vi "VisionOnSWMap5LabModifiedOne.vi"(0 "SWMap In":i32[][](array[numeric]), 11 "Image Pixels":u32[][](array[numeric])) -> (4 "SWMap Out":i32[][](array[numeric]))   [LabVIEW 2014]
panel:
  out "test3":dbl
  out "test2":dbl
  out "test1":dbl
  # "Vision On SWMap"
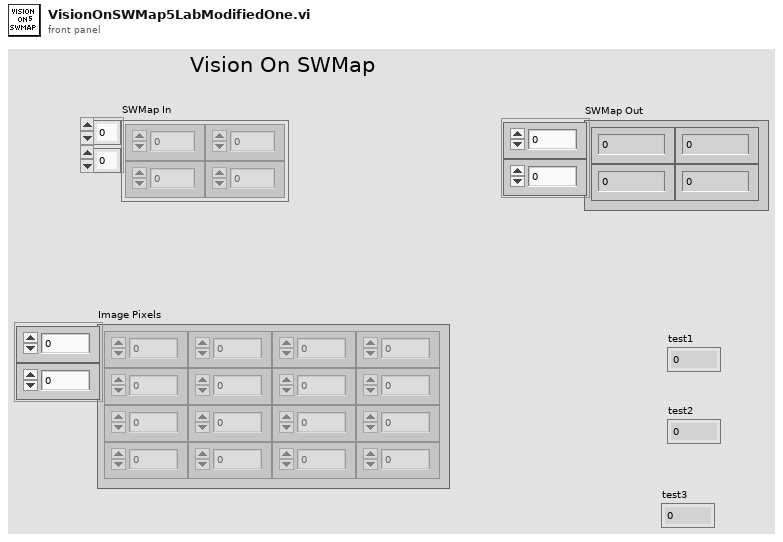
[diagram p1: front panel]
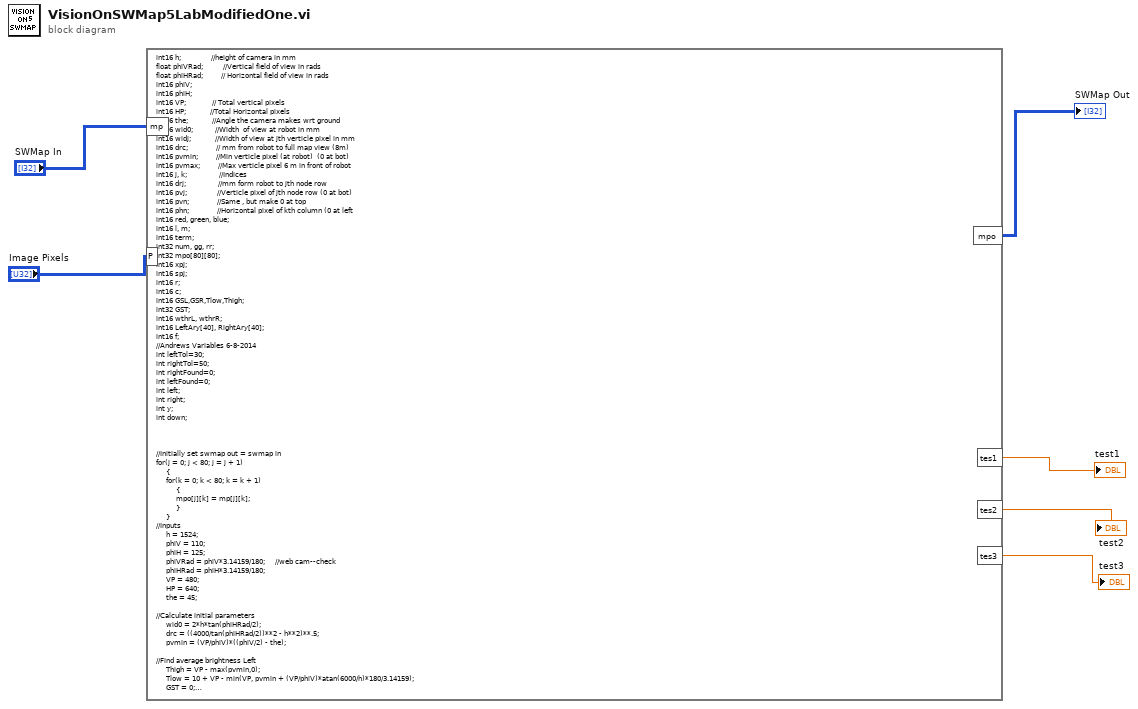
[diagram p0: block diagram]
diagram:
  n1 = formula code="int16 h;               //height of camera in mm\nfloat phiVRad;          //Vertical field of view in rads\nfloat phiHRad;         // Horizontal field of view in rads\nint16 phiV;\nint16 phiH;\nint16 VP;             // Total vertical pixels\nint16 HP;            //Total Horizontal pixels\nint16 the;            //Angle the camera makes wrt ground\nint16 wid0;           //Width  of view at robot in mm\nint16 widj;            //Width of view at jth verticle pixel in mm\nint16 drc;              // mm from robot to full map view (8m)\nint16 pvmin;         //Min verticle pixel (at robot)  (0 at bot)\nint16 pvmax;         //Max verticle pixel 6 m in front of robot\nint16 j, k;                //Indices\nint16 drj;                //mm form robot to jth node row\nint16 pvj;               //Verticle pixel of jth node row (0 at bot)\nint16 pvn;              //Same , but make 0 at top\nint16 phn;              //Horizontal pixel of kth column (0 at left\nint16 red, green, blue;\nint16 l, m;\nint16 term;\nint32 num, gg, rr;\nint32 mpo[80][80];\nint16 xpj;\nint16 spj;\nint16 r;\nint16 c;\nint16 GSL,GSR,Tlow,Thigh;\nint32 GST;\nint16 wthrL, wthrR;\nint16 LeftAry[40], RightAry[40];\nint16 f;\n//Andrews Variables 6-8-2014\nint leftTol=30;\nint rightTol=50;\nint rightFound=0;\nint leftFound=0;\nint left;\nint right;\nint y;\nint down;\n\n\n\n//Initially set swmap out = swmap in\nfor(j = 0; j < 80; j = j + 1)\n     {\n     for(k = 0; k < 80; k = k + 1)\n          {\n          mpo[j][k] = mp[j][k];\n          }\n     }\n//Inputs\n     h = 1524;\n     phiV = 110;\n     phiH = 125;\n     phiVRad = phiV*3.14159/180;     //web cam--check\n     phiHRad = phiH*3.14159/180;\n     VP = 480;\n     HP = 640;\n     the = 45;  \n\n//Calculate initial parameters\n     wid0 = 2*h*tan(phiHRad/2);   \n     drc = ((4000/tan(phiHRad/2))**2 - h**2)**.5;\n     pvmin = (VP/phiV)*((phiV/2) - the);\n\n//Find average brightness Left\n     Thigh = VP - max(pvmin,0);\n     Tlow = 10 + VP - min(VP, pvmin + (VP/phiV)*atan(6000/h)*180/3.14159);\n     GST = 0;\n     for(l = Tlow;l < Thigh;l = l + 10)\n          {\n               for(m = 10;m < HP/2;m = m + 10)\n                    {\n                         num = P[l][m];\n                         blue = num % 256;\n                         gg = (num - blue)/256;\n                         green = gg % 256;\n                         rr = num - blue - (green * 256);\n                         red = rr/(256 * 256);\n                         GST = GST + (red + green + blue)/3;\n                    }\n            }\n      GSL = GST/(((VP/10) - 1) * ((HP/20) - 1));\n\n//Find average brightness Right\n     GST = 0;\n     for(l = Tlow;l < Thigh;l = l + 10)\n          {\n               for(m = 10 + HP/2 ; m < HP ; m = m + 10)\n                    {\n                         num = P[l][m];\n                         blue = num % 256;\n                         gg = (num - blue)/256;\n                         green = gg % 256;\n                         rr = num - blue - (green * 256);\n                         red = rr/(256 * 256);\n                         GST = GST + (red + green + blue)/3;\n                    }\n            }\n      GSR = GST/(((VP/10) - 1) * ((HP/20) - 1));\n\n//Find white threshold based on brightness\n     wthrL = min(GSL + 60, 255);\n     wthrR = min(GSR + 60, 255); \n\ntes1 = GSL;\ntes2 = wthrL;\ntes3 = wthrR;\n\n//Adjust max verticle node based on drc\n     if(drc > 6000)\n          {term = 6000;}\n     else\n          {term = drc;}\n\n//Loop thru each node in camera's view to find pixels\n     j = 60;\n     while( j > 60 - term/100 - 1)   //from robot to drc line\n     {\n          widj = (((wid0 -8000)*100*(j - 60))/drc) + wid0;\n          drj = 6000 - (100 * j);\n          pvj = pvmin + (VP/phiV)*atan(drj/h)*180/3.14159;\n                   \n          if(pvj > 0 && pvj < VP)\n          {\n               pvn = VP - pvj;\n               if(pvn < 1)\n                    {pvn = 1;}\n               if(pvn > VP-2)\n                    {pvn = VP - 2;}\n               k = 40 - widj/200;\n              \n               while(k < (41 +widj/200))\n               {\n                    phn = (k - 40 + widj/200) * (HP * 100) / widj;\n                    if(phn < 1)\n                         {phn = 1;}\n                    if(phn > HP-2)\n                         {phn = HP - 2;}\n                    red = 0;\n                    green = 0;\n                    blue = 0;\n\n                   l = -1;\n                   while(l <2)\n                   {\n                        m = -1; \n                        while(m < 2)\n                        {\n                             num = P[pvn + m][phn + l];\n                             blue = blue + num % 256;\n                             gg = (num - (num % 256)) / 256;\n                             green = green + gg % 256;\n                             rr = num - (num % 256) - ((gg % 256) * 256);\n                             red = red + rr/(256 * 256);\n                             m = m + 1;\n                         }\n\n                         l = l + 1;\n                    }\n                    red = red/9;\n                    green = green/9;\n                    blue = blue/9;\n                    if(mpo[j][k] == 1000)\n                    {\n                         if(k <= HP/2)\n                              {\n                                   if (red > wthrL && green > wthrL && blue > wthrL)\n                                        {mpo[j][k] = 3500;}\n                              } \n                         if(k > HP/2)\n                              {\n                                   if (red > wthrR && green > wthrR && blue > wthrR)\n                                        {mpo[j][k] = 3500;}\n                              } \n                         if(red - green > 50 && red - blue > 50)\n                              {mpo[j][k] = 4000;}\n                         if(blue - green > 50 && blue - red > 50)\n                              {mpo[j][k] = 4500;}\n                    }\n\n                    \n                    k = k + 1;\n               }\n          }\n          j = j-1;\n     }\n//Next do from drc line to top of 8 x 8 meter map\n     if(term < 6000)  //only for large FOV cameras\n     {\n          while(j > -1)     //from drc line to top\n          {\n              drj = 6000 - (100 * j);\n              pvj = pvmin + (VP/phiV)*atan(drj/h)*180/3.14159;\n              widj = 2 * ((h**2 + drj**2)**.5) * tan(phiHRad/2);\n              pvn = VP - pvj;\n               if(pvn < 1)\n                    {pvn = 1;}\n               xpj = HP * (8000/widj);     //num of pixels across all 80 nodes at row j\n               spj = (HP/2) - (xpj/2);       //num of pixels to left of 80x80\n               k = 0;\n               while(k < 80)\n               {\n                    phn = spj + (xpj/80) * k;\n                    if(phn < 1)\n                         {phn = 1;}\n                    if(phn > HP-2)\n                         {phn = HP - 2;}\n                    red = 0;\n                    green = 0;\n                    blue = 0;\n                    l = -1;\n                    while(l <2)\n                    {\n                         m = -1; \n                         while(m < 2)\n                         {\n                              num = P[pvn + m][phn + l];\n                              blue = blue + num % 256;\n                              gg = (num - (num % 256)) / 256;\n                              green = green + gg % 256;\n                              rr = num - (num % 256) - ((gg % 256) * 256);\n                              red = red + rr/(256 * 256);\n                              m = m + 1;\n                         }\n                         l = l + 1;\n                    }\n                    red = red/9;\n                    green = green/9;\n                    blue = blue/9;\n                    if(mpo[j][k] == 1000)\n                    {\n                         if(k <= HP/2)\n                              {\n                                   if (red > wthrL && green > wthrL && blue > wthrL)\n                                        {mpo[j][k] = 3500;}\n                              } \n                         if(k > HP/2)\n                              {\n                                   if (red > wthrR && green > wthrR && blue > wthrR)\n                                        {mpo[j][k] = 3500;}\n                              } \n\n                         if(red - green > 50 && red - blue > 50)\n                              {mpo[j][k] = 4000;}\n                         if(blue - green > 50 && blue - red > 50)\n                              {mpo[j][k] = 4500;}\n                    }\n                    k = k + 1;\n               }\n               j = j-1;\n          }\n     }\n\n//Algorithm for Color Expansion\n//begin outer for loop\n      for(r = 0; r < 80; r++){\n          //begin nested for loop\n               for(c = 0; c < 80; c++){\n                    if(mpo[r][c] == 3500 || mpo[r][c] == 4000 || mpo[r][c] == 4500){//encasing if statement\n                         if(c-1 >= 0){//left check\n                              if(mpo[r][c-1] != 3500 && mpo[r][c-1] != 4000 && mpo[r][c-1] != 4500 && mpo[r][c-1] != 2500)\n                                   {mpo[r][c-1] += 100;}\n                             \tif(r-1 >= 0){\n                                   if(mpo[r-1][c-1] != 3500 && mpo[r-1][c-1] != 4000 && mpo[r-1][c-1] != 4500 && mpo[r-1][c-1] != 2500)\n                                       \t{mpo[r-1][c-1] += 100;}\n                                   }\n                              if(r+1 <= 79){\n                                   if(mpo[r+1][c-1] != 3500 && mpo[r+1][c-1] != 4000 && mpo[r+1][c-1] != 4500 && mpo[r+1][c-1] != 2500)\n                                        {mpo[r+1][c-1] +=100;}\n                              }//end subsequent checks (nested, part of the left if statement check structure\t\n                         }//end left check\n                        \tif(r-1 >= 0){ //top check\n                             \tif(mpo[r-1][c] != 3500 && mpo[r-1][c] != 4000 && mpo[r-1][c] != 4500 && mpo[r-1][c] != 2500)\n                                  {mpo[r-1][c] += 100;}\n                         }//end top check: r-1\n                        \tif(r+1 <= 79){//bottom check\n                                   if(mpo[r+1][c] != 3500 && mpo[r+1][c] != 4000 && mpo[r+1][c] != 4500 && mpo[r+1][c] != 2500)\n                                        {mpo[r+1][c] += 100;}\n                         }//end bottom check: r+1\n                         if(c+1 <=79){//right check\n                              if(mpo[r][c+1] != 3500 && mpo[r][c+1] != 4000 && mpo[r][c+1] != 4500 && mpo[r][c+1] != 2500)\n                                   {mpo[r][c+1] += 100;}\n                              if(r-1 >= 0){\n                                   if(mpo[r-1][c+1] != 3500 && mpo[r-1][c+1] != 4000 && mpo[r-1][c+1] != 4500 && mpo[r-1][c+1] != 2500)\n                                        {mpo[r-1][c+1] += 100;}\n                              }//end nested if stmt 1\n                             \tif(r+1 <= 79){\n                                   if(mpo[r+1][c+1] != 3500 && mpo[r+1][c+1] != 4000 && mpo[r+1][c+1] != 4500 && mpo[r+1][c+1] != 2500)\n                                        {mpo[r+1][c+1] += 100;}\n                           }//end r+1 check (nested if stmt)\n                         }//end right check\n                    }//end encasing if statement\n            }//end nested for loop\n      }//end outer for loop\n\n//Next is Andrew and Hollie's code for adding lines and filling the spaces outside the lines\n/*\n//initialize both arrays to be filled w/ the value -1:\n     for(j=0; j < 40; j = j + 1)\n          {\n                LeftAry[j] = -1;\n                RightAry[j] = -1;\n          }\nfor(j = 79; j>= 0; j = j - 1){ //OPENING BRACE FOR j LOOP (up and down)\n\tfor(k = 0; k <= 39; k = k + 1){ //OPENING BRACE FOR k LOOP (left to right)\n\t\tif(mpo[j][k] == 3500 || mpo[j][k] == 3600){ //OPENING: IF\n\t\t\tLeftAry[j] = k;\n   break;\n\t\t} //CLOSING BRACE: IF STATEMENT\n\t} //CLOSING BRACE: k LOOP (left to right)\n\tfor(k = 79; k >= 40; k = k - 1){ //OPENING BRACE FOR k LOOP (right to left)\n\t\tif(mpo[j][k] == 3500 || mpo[j][k] == 3600){ //OPENING: IF\n\t\t\tRightAry[j] = k;\n   break;\n\t\t} //CLOSING BRACE: IF STATEMENT\n\t} //CLOSING BRACE: k LOOP (right to left)\n} //CLOSING BRACE: j LOOP (up and down)\n\n//LOGIC SHIFT\nfor(j= 79; j >= 0; j = j - 1){ //OPENING BRACE FOR K LOOP (up and down)\n\tif(LeftAry[j] == -1 && RightAry[j] == -1){ \n\t\tmpo[j][24] = 3700;\n\t\tmpo[j][55] = 3700;\n\n\t} \n\n\tif(LeftAry[j] != -1 && RightAry[j] == -1){ \n\t\tmpo[j][k+31] = 3700; //Generate white, make new color, fill loop.\n\t} //CLOSING BRACE:  IF STMT FOR LWHITE !RWHITE\n\tif(LeftAry[j] == -1 && RightAry[j] != -1){ //RIGHT WHITE, no LEFT WHITE\n\t\tmpo[j][k-31] == 3700; //Generate white, make new color, fill loop\n\t} //CLOSING BRACE:  IF STMT FOR RWHITE !LWHITE\t\n\n\tfor(f = RightAry[k]; f < 79; f = f + 1){ //OPENING BRACE FOR F LOOP\n\t\tmpo[j][f+1] = 3700;\n\t} //CLOSING BRACE FOR F LOOP\n\tfor(f = LeftAry[j]; f > 0; f = f - 1){ //OPENING BRACE FOR F LOOP\n\t\tmpo[j][f-1] = 3700;\n\t} //CLOSING BRACE FOR F LOOP\n}//CLOSING BRACE: K LOOP\ntes1 = 555;\n*/\n\n\nfor ( y=0;y<80;y=y+1){\n//LEFT SIDE LINE CREATION\n    for( left=0;left<=leftTol;left=left+1){\n         if(mpo[y][left]!=3500&&mpo[y][left]!=2500){\n              mpo[y][left]=3500;\n         }else if(mpo[y][left]==1&&leftFound==0){\n            leftFound=1;\n            for( down=y+1;down<=79;down=down+1){\n                 if(mpo[down][left]!=2500){\n                     mpo[down][left]=3500;\n                  }\n             } \n             break;   \n         }else{\n            break;\n         }\n    }\n      //RIGHT SIDE CREATION\n       for( right=79;right>=rightTol;right=right-1){\n         if(mpo[y][right]!=3500&&mpo[y][right]!=2500){\n              mpo[y][right]=3500;\n         }else if(mpo[y][right]==1&&rightFound==0){\n            rightFound=1;\n            for( down=y+1;down<=79;down=down+1){\n                 if(mpo[down][right]!=2500){\n                     mpo[down][right]=3500;\n                  }\n             } \n             break;   \n         }else{\n            break;\n         }\n    }\n}\n\n\n\n\n\n\n\n//Erase the front of the robot\nfor (j = 54; j < 61;j = j + 1)\n     {\n          for (k = 34; k < 47; k = k + 1)\n      {mpo[j][k] = 1000;\n}\n     }"("P"="Image Pixels", "mp"="SWMap In") -> ("mpo"=→"SWMap Out":i32[][], "tes1"=→"test1":dbl, "tes2"=→"test2":dbl, "tes3"=→"test3":dbl)
